vi "Separate_Times.vi"(11 "Frame":string) -> (2 "Base Time":T1 {"HIGH" max=10 step=1; "MEDIUM" max=10 step=1; "LOW" max=10 step=1; "DELICATE" max=10 step=1}, 3 "Increment Time":T1 {"HIGH" max=10 step=1; "MEDIUM" max=10 step=1; "LOW" max=10 step=1; "DELICATE" max=10 step=1})   [LabVIEW 2023]
panel:
  out "error out":errorcluster
  in  "error in":errorcluster
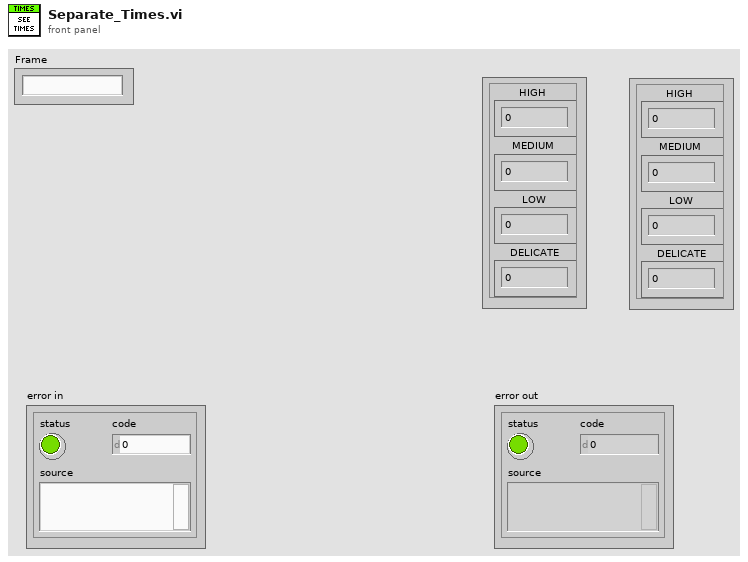
[diagram p1: front panel]
types:
  T1 = cluster{"DELICATE":u32, "LOW":u32, "MEDIUM":u32, "HIGH":u32}
  T2 = cluster{"Delicates":u32, "Low":u32, "Medium":u32, "High":u32}
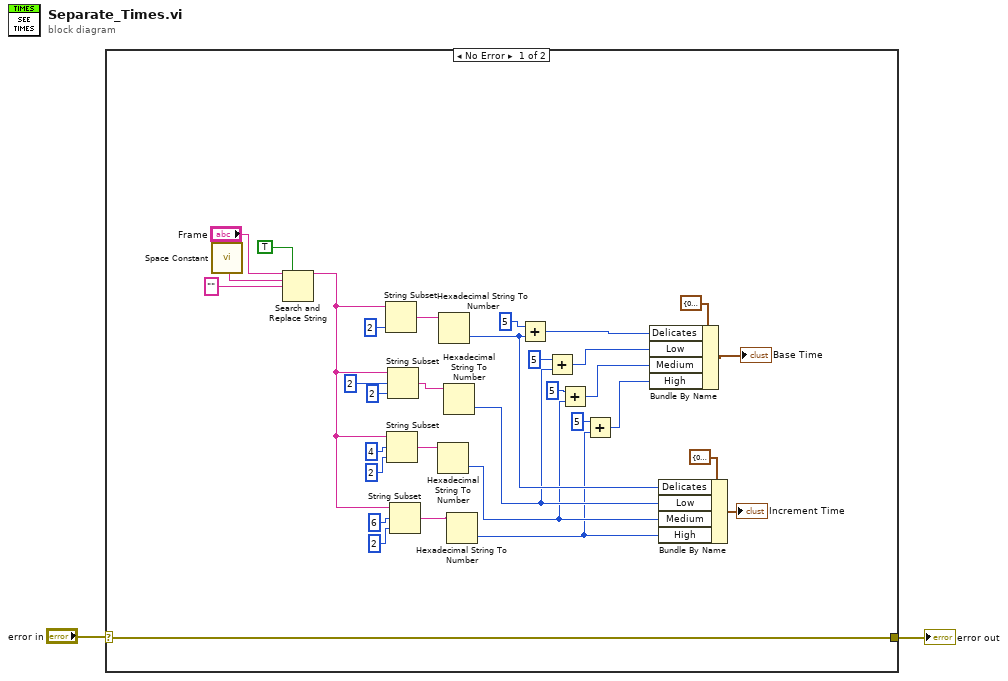
[diagram p0: block diagram]
diagram:
  n1 = case shown="No Error" "error in" {
    selector: "error in" -> [w22 w36]
    tunnel: [w22 w36] -> w1
    frame No Error {
      n2 = call <vilib>:"Space Constant.vi"() -> ("String"=w32:string)
      n3 = Search and Replace String(replace all?=TRUE ("replace all? (F)"), input string="Frame", search string=w32, replace string="" ("replace string (\"\")")) -> (result string=w24:string)  [unwired: 4 in, 3 out]
      n4 = String Subset(string=w24, length (rest)=2 ("length (rest)")) -> (substring=w21:string)  [unwired: 1 in]
      n5 = String Subset(string=w24, offset (0)=4, length (rest)=2 ("length (rest)")) -> (substring=w19:string)
      n6 = String Subset(string=w24, offset (0)=2, length (rest)=2 ("length (rest)")) -> (substring=w20:string)
      n7 = String Subset(string=w24, offset (0)=6, length (rest)=2 ("length (rest)")) -> (substring=w18:string)
      n8 = Hexadecimal String To Number(string=w19) -> (number=w11:u32)  [unwired: 2 in, 1 out]
      n9 = Hexadecimal String To Number(string=w21) -> (number=w16:u32)  [unwired: 2 in, 1 out]
      n10 = Hexadecimal String To Number(string=w20) -> (number=w13:u32)  [unwired: 2 in, 1 out]
      n11 = Hexadecimal String To Number(string=w18) -> (number=w9:u32)  [unwired: 2 in, 1 out]
      n12 = Add(x=u32 5, y=w16) -> (x+y=w7:u32)
      n13 = Add(x=u32 5, y=w13) -> (x+y=w6:u32)
      n14 = Add(x=u32 5, y=w11) -> (x+y=w5:u32)
      n15 = Add(x=u32 5, y=w9) -> (x+y=w4:u32)
      n16 = Bundle By Name(cluster=T2 {"Delicates"=0, "Low"=0, "Medium"=0, "High"=0}, "Delicates"=w7, "Low"=w6, "Medium"=w5, "High"=w4) -> (→"Base Time":T2)
      n17 = Bundle By Name(cluster=T2 {"Delicates"=0, "Low"=0, "Medium"=0, "High"=0}, "Delicates"=w16, "Low"=w13, "Medium"=w11, "High"=w9) -> (→"Increment Time":T2)
    }
    frame Error {
    }
  }
  "error out" <- w1
